vi "状态判断.vi"(0 "数值":u8) -> (1 "D0":bool, 2 "D01":bool, 3 "D02":bool)   [LabVIEW 2012]
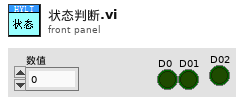
[diagram p1: front panel]
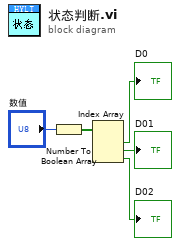
[diagram p0: block diagram]
diagram:
  n1 = Number To Boolean Array(number="数值") -> (Boolean array=w4:bool[])
  n2 = Index Array(array=w4) -> (element #1=→"D0":bool, element #2=→"D01":bool, element #3=→"D02":bool)  [unwired: 3 in]
